vi "Commands.vi"() -> (0 "Commands":T1[](array[typedef])=["Stop", "Set Channel", "CONTROL:DLConnect", "CONTROL:DLConnected", "CONTROL:DetConnect", "CONTROL:DetConnected", "CONTROL:DAQmxConnect", "CONTROL:DAQmxConnected", "CONTROL:OScConnect", "CONTROL:OScConnected", "CONTROL:AllConnect", "CONTROL:Status", "DL:MoveAxis", "DL:MovedAxis", "DET:Read", "DET:ReadDONE", "DAQmx:MoveCrystal", "DAQmx:MovedCrystal", "DAQmx:AcceleratorShutter", "DAQmx:AcceleratorShutterDONE", "DAQmx:LaserShutter", "DAQmx:LaserShutterDONE", "DAQmx:RelayKeyHeater", "DAQmx:RelayKeyHeaterDONE", "DAQmx:LaserShutterDONE", "DAQmx:HeaterAlarm", "DAQmx:PowerStatus", "DAQmx:FaradayCupStatus", "DAQmx:FaradayCup", "DAQmx:FaradayCupDONE", "OSc:Read", "OSc:ReadDONE", "Error", "DAQmx:ELYSE_pulse_counter"])   [LabVIEW 2020]
uses:
  <vilib>/NI/STM/SubVIs/MetaDataElement.ctl
  <vilib>/NI/STM/NI STM.lvlib
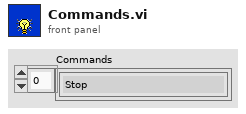
[diagram p1: front panel]
types:
  T1 = typedef "NI STM.lvlib/MetaDataElement.ctl" = string
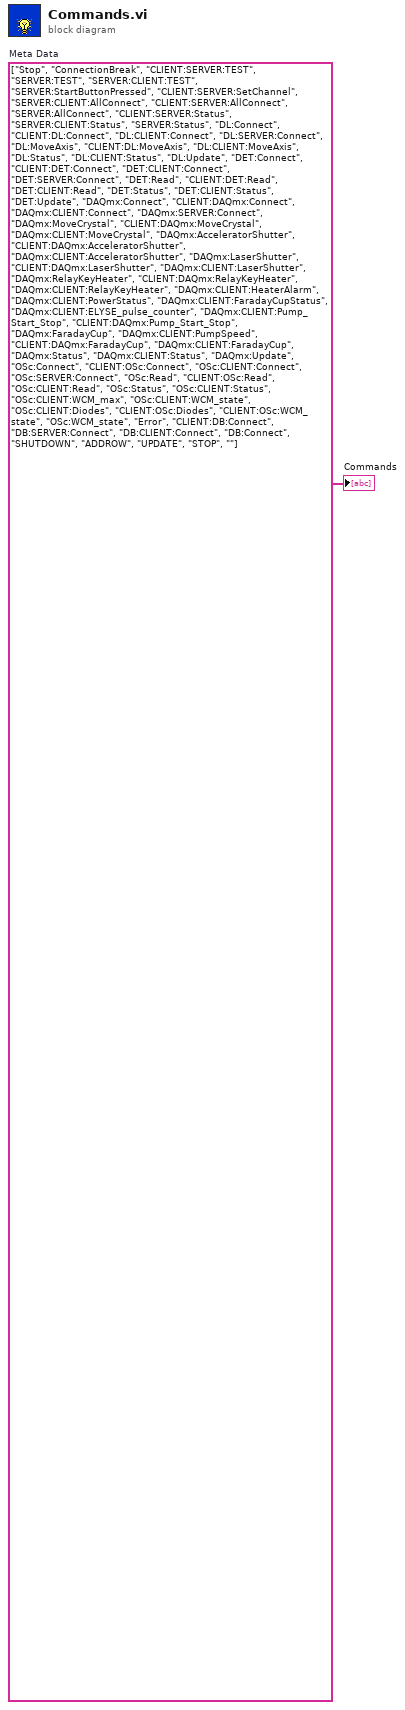
[diagram p0: block diagram]
diagram:
  w1 = T1[] ["Stop", "ConnectionBreak", "CLIENT:SERVER:TEST", "SERVER:TEST", "SERVER:CLIENT:TEST", "SERVER:StartButtonPressed", "CLIENT:SERVER:SetChannel", "SERVER:CLIENT:AllConnect", "CLIENT:SERVER:AllConnect", "SERVER:AllConnect", "CLIENT:SERVER:Status", "SERVER:CLIENT:Status", "SERVER:Status", "DL:Connect", "CLIENT:DL:Connect", "DL:CLIENT:Connect", "DL:SERVER:Connect", "DL:MoveAxis", "CLIENT:DL:MoveAxis", "DL:CLIENT:MoveAxis", "DL:Status", "DL:CLIENT:Status", "DL:Update", "DET:Connect", "CLIENT:DET:Connect", "DET:CLIENT:Connect", "DET:SERVER:Connect", "DET:Read", "CLIENT:DET:Read", "DET:CLIENT:Read", "DET:Status", "DET:CLIENT:Status", "DET:Update", "DAQmx:Connect", "CLIENT:DAQmx:Connect", "DAQmx:CLIENT:Connect", "DAQmx:SERVER:Connect", "DAQmx:MoveCrystal", "CLIENT:DAQmx:MoveCrystal", "DAQmx:CLIENT:MoveCrystal", "DAQmx:AcceleratorShutter", "CLIENT:DAQmx:AcceleratorShutter", "DAQmx:CLIENT:AcceleratorShutter", "DAQmx:LaserShutter", "CLIENT:DAQmx:LaserShutter", "DAQmx:CLIENT:LaserShutter", "DAQmx:RelayKeyHeater", "CLIENT:DAQmx:RelayKeyHeater", "DAQmx:CLIENT:RelayKeyHeater", "DAQmx:CLIENT:HeaterAlarm", "DAQmx:CLIENT:PowerStatus", "DAQmx:CLIENT:FaradayCupStatus", "DAQmx:CLIENT:ELYSE_pulse_counter", "DAQmx:CLIENT:Pump_Start_Stop", "CLIENT:DAQmx:Pump_Start_Stop", "DAQmx:FaradayCup", "DAQmx:CLIENT:PumpSpeed", "CLIENT:DAQmx:FaradayCup", "DAQmx:CLIENT:FaradayCup", "DAQmx:Status", "DAQmx:CLIENT:Status", "DAQmx:Update", "OSc:Connect", "CLIENT:OSc:Connect", "OSc:CLIENT:Connect", "OSc:SERVER:Connect", "OSc:Read", "CLIENT:OSc:Read", "OSc:CLIENT:Read", "OSc:Status", "OSc:CLIENT:Status", "OSc:CLIENT:WCM_max", "OSc:CLIENT:WCM_state", "OSc:CLIENT:Diodes", "CLIENT:OSc:Diodes", "CLIENT:OSc:WCM_state", "OSc:WCM_state", "Error", "CLIENT:DB:Connect", "DB:SERVER:Connect", "DB:CLIENT:Connect", "DB:Connect", "SHUTDOWN", "ADDROW", "UPDATE", "STOP", ""]  # Meta Data
  "Commands" <- w1
